vi "Write Config Unitest.vi"(8 "error in (no error)":errorcluster, 11 "main ref":T1) -> (0 "error out":errorcluster)   [LabVIEW 2025]
uses:
  v06/controls/LAB-IQ UI Data.ctl
  Traction Loop/Traction Receipe Enum.ctl
  Config file  FGV Unitest enum.ctl
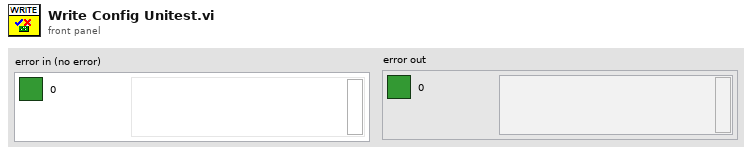
[diagram p1: front panel]
types:
  T1 = typedef "LAB-IQ UI Data.ctl" = cluster{"Main Home Screen":cluster{"GUI":refnum<vi>, "Platform Settings":refnum<vi>, "Configure":refnum<vi>, "Home":refnum<vi>, "EXIT":refnum<vi>, "service 2":refnum<vi>, "MainPage":refnum<vi>, "Analysis":refnum<vi>}, "Platform Settings":cluster{"mm/s  Surge":refnum<vi>, "Drive Error":refnum<vi>, "Disable Axis Jog Soft Limits":refnum<vi>, "mm/s  Sway":refnum<vi>, "Sway and Surge COM Status":refnum<vi>, "Heave COM Status":refnum<vi>, "Enable Platform":refnum<vi>, "Surge Forward Main":refnum<vi>, "Sway Right Main":refnum<vi>, "Sway Left Main":refnum<vi>, "Heave Down Main":refnum<vi>, "Heave Up main":refnum<vi>, "mm/s Heave":refnum<vi>, "mm/sec":refnum<vi>, "mm":refnum<vi>, "Surge Backward Main":refnum<vi>}, "Analysis Screen":cluster{"Analysis Home":refnum<vi>, "Surface Analysis":refnum<vi>, "Imaging":refnum<vi>, "Image Analysis":refnum<vi>, "Post Analysis":refnum<vi>}, "Config Screen":cluster{"Select Load Head":refnum<vi>, "Notes :":refnum<vi>, "FILE":refnum<vi>, "Sample ID :":refnum<vi>, "Operator ID :":refnum<vi>, "Operator Name :":refnum<vi>, "Auto":refnum<vi>}, "Motion Module":cluster{"zNL":refnum<vi>, "NL disp":refnum<vi>, "Rotary Tab":refnum<vi>, "Motion Direction:  3":refnum<vi>, "E.Velocity 2":refnum<vi>, "e.v/ssr 2":refnum<vi>, "Enter Fixed E.Velocity 2":refnum<vi>, "Enter Final SRR 2":refnum<vi>, "Enter initial SRR 2":refnum<vi>, "Enter Fixed SRR 2":refnum<vi>, "Enter the Final E.Velocity (m/s) 2":refnum<vi>, "Enter initial E.Velocity (m/s) 2":refnum<vi>, "Final Speed (RPM) 3":refnum<vi>, "Initial Speed (RPM) 2":refnum<vi>, "Enter the Final Velocity (m/s) 3":refnum<vi>, "Enter initial Velocity (m/s)  3":refnum<vi>, "Ramp Up 2":refnum<vi>, "TEST SELECTION":refnum<vi>, "SPEED SELECTION : ":refnum<vi>, "Angular Oscillation Set":refnum<vi>, "Traction":refnum<vi>, "Step Speed":refnum<vi>, "StepTable For Load-Speed":refnum<vi>, "StepTable For Speed":refnum<vi>, "Surge Forward MM":refnum<vi>, "Surge Backward MM":refnum<vi>, "M3 Image":refnum<vi>, "String 39":refnum<vi>, "Sway Left MM":refnum<vi>, "Sway Right MM":refnum<vi>, "Disable Axis Jog Soft Limits":refnum<vi>, "mm":refnum<vi>, "Heave Down MM":refnum<vi>, "Heave Up MM":refnum<vi>, "Wear Track Diameter (mm)":refnum<vi>, "Set WTD":refnum<vi>, "HomeScratch":refnum<vi>, "HomeRot":refnum<vi>, "PlaceModule":refnum<vi>, "Enter the Angle (Deg)":refnum<vi>, "Enter the Frequency (Hz)":refnum<vi>, "Motion Mode:":refnum<vi>, "LR Sway":refnum<vi>, "Rot Hor":refnum<vi>, "Scratch":refnum<vi>, "LR Cam":refnum<vi>, "MMBack":refnum<vi>, "MMNext":refnum<vi>, "Rot Ver":refnum<vi>, "Rotary Module Selection":refnum<vi>, "calculate rotary":refnum<vi>, "SPEED SELECTION : rotary":refnum<vi>, "Import 2":refnum<vi>, "Save 2":refnum<vi>, "File Path :  2":refnum<vi>, "String 45":refnum<vi>, "StepTable For Speed 3":refnum<vi>, "Enter the Speed(mm/sec)":refnum<vi>, "Enter the Speed(RPM)":refnum<vi>, "Enter Scratch Speed (mm/s):":refnum<vi>, "SwaySpeed Set":refnum<vi>, "Scartch Offset":refnum<vi>, "Motion type:":refnum<vi>, "HomeScratch 2":refnum<vi>, "Enter Scratch length (mm):":refnum<vi>, "Wear Track Diameter":refnum<vi>, "Rotary Speed Exced":refnum<vi>, "Scratch Mode":refnum<vi>, "No of Scratch":refnum<vi>}, "Environmental control":cluster{"Humidity  Status  3":refnum<vi>, "Low Temp  Status  2":refnum<vi>, "TK4 status 2":refnum<vi>, "Stage Temperature":refnum<vi>, "Sample Temperature":refnum<vi>, "Humidity (Amb)":refnum<vi>, "Clear List":refnum<vi>, "Add to list":refnum<vi>, "Wear":refnum<vi>, "Vibration":refnum<vi>, "Humidity (Chamber)":refnum<vi>, "Temperature (Chamber)":refnum<vi>, "ECR ":refnum<vi>, "Temperature (Amb)":refnum<vi>, "Microphone":refnum<vi>, "Acoustic Emission 3":refnum<vi>, "SNext":refnum<vi>, "APBack":refnum<vi>, "Enter the Temperature (°C):":refnum<vi>, "Enter the Stage \nTemperature (°C):":refnum<vi>, "Enter the Humidity (%Rh):":refnum<vi>, "Low Temp":refnum<vi>, "High Temp":refnum<vi>, "Humidity":refnum<vi>, "Sensors Picked":refnum<vi>}, "About Screen":cluster{"Password":refnum<vi>, "Home Service":refnum<vi>, "Advanced Setting":refnum<vi>, "About Tab":refnum<vi>, "ECR Port:":refnum<vi>, "Ramp Port:":refnum<vi>, "Installation/Replacement completed":refnum<vi>, "Loahead":refnum<vi>, "Heave and Surge COM Port:":refnum<vi>, "Sway COM Port:":refnum<vi>, "Temp Modbus:":refnum<vi>, "Humidity Port:":refnum<vi>, "Edit Gain Constants":refnum<vi>, "Save Gain Constants":refnum<vi>}, "Main Screen":cluster{"Main Screen Tab":refnum<vi>, "Angle and Frequency":refnum<vi>, "Stroke (mm)":refnum<vi>, "Angle (Deg)":refnum<vi>, "Main Speed Tab":refnum<vi>, "MTM MOTOR DISPLAY":refnum<vi>, "Disc Speed (m/sec)":refnum<vi>, "Ball Speed (m/sec)":refnum<vi>, "Disc Speed (RPM)":refnum<vi>, "Ball Speed (RPM)":refnum<vi>, "SPEED TAB":refnum<vi>, "Speed (m/sec)":refnum<vi>, "Set Speed (m/sec)":refnum<vi>, "Speed (RPM)":refnum<vi>, "Set Speed":refnum<vi>, "Time Tab":refnum<vi>, "Time ( HH:MM:SS ) 2":refnum<vi>, "Test Duration":refnum<vi>, "Test Duration 4":refnum<vi>, "TEST CYCLE":refnum<vi>, "TOTAL CYCLES":refnum<vi>, "Set Load (N)":refnum<vi>, "Temp Tabs":refnum<vi>, "Heater":refnum<vi>, "TK4 status":refnum<vi>, "ChamberTemp":refnum<vi>, "SetTmp":refnum<vi>, "Controller  Status":refnum<vi>, "ChamberTemp 2":refnum<vi>, "SetTmp 2":refnum<vi>, "Controller  Status 2":refnum<vi>, "ChamberTemp 3":refnum<vi>, "SetTmp 3":refnum<vi>, "Cooling":refnum<vi>, "Load Communication":refnum<vi>, "Ambient \nTemperature":refnum<vi>, "HumCOMStatus":refnum<vi>, "Ambient\n Humidity":refnum<vi>, "Freq (Hz)":refnum<vi>, "Load En":refnum<vi>, "NLt":refnum<vi>, "zNL 2":refnum<vi>, "Humidity On":refnum<vi>, "humidity disp":refnum<vi>, "Set Humidity":refnum<vi>, "NL disp 2":refnum<vi>, "Humidity On 2":refnum<vi>, "humidity disp 2":refnum<vi>, "Set Humidity 2":refnum<vi>, "NL disp 3":refnum<vi>, "AppLoadSeq scratch":refnum<vi>, "Stop Scratch":refnum<vi>, "ClrLog":refnum<vi>, "Trip Log":refnum<vi>, "STOP":refnum<vi>, "Start Test":refnum<vi>, "Test status":refnum<vi>, "AR Led":refnum<vi>, "Data":refnum<vi>, "Health":refnum<vi>, "Sway COM Status":refnum<vi>, "Heave COM Status":refnum<vi>, "Grp Tab":refnum<vi>, "Sub Graph":refnum<vi>, "SD (mm)":refnum<vi>, "Siliding distance Reset Graph":refnum<vi>, "SDGp":refnum<vi>, "Humidity Reset Graph":refnum<vi>, "HumrGp":refnum<vi>, "Acoustic Emission (mV)":refnum<vi>, "Aqucostic Reset Graph":refnum<vi>, "gACQUOS":refnum<vi>, "ECR RESET":refnum<vi>, "ECR":refnum<vi>, "Temperature Reset":refnum<vi>, "Acoustic Emission (mV) 2":refnum<vi>, "Aqucostic Reset Graph 2":refnum<vi>, "gACQUOS 2":refnum<vi>, "ECR RESET 2":refnum<vi>, "ECR 2":refnum<vi>, "Temperature Reset 2":refnum<vi>, "Temperature (deg c)":refnum<vi>, "Speed Reset Graph":refnum<vi>, "Speed Tab":refnum<vi>, "MTM DISC  SPEED":refnum<vi>, "MTM BALL SPEED":refnum<vi>, "speed mm/sec":refnum<vi>, "Hymidity":refnum<vi>, "Humidity Disable trip":refnum<vi>, "CoF Trip  2":refnum<vi>, "Depth Trip":refnum<vi>, "Weart Deapth":refnum<vi>, "Depth Reset Graph":refnum<vi>, "Weart":refnum<vi>, "Depthz":refnum<vi>, "Depth (µm)":refnum<vi>, "WearGp":refnum<vi>, "NL Trip 2":refnum<vi>, "Load pid":refnum<vi>, "Load Disable Trip":refnum<vi>, "Load Reset Graph":refnum<vi>, "NL Display 4":refnum<vi>, "Main Chart 3":refnum<vi>, "BACK":refnum<vi>, "Depth Trip 2":refnum<vi>, "COF TRIP ":refnum<vi>, "Friction Force (N)":refnum<vi>, "FF Reset Graph":refnum<vi>, "FF Disable Trip":refnum<vi>, "FF TRIP":refnum<vi>, "COF Disable Trip":refnum<vi>, "COF Reset Graph":refnum<vi>, "Start Test Temp":refnum<vi>, "zFF":refnum<vi>, "Friction Force (N) Graph":refnum<vi>, "Coefficient of Friction":refnum<vi>, "Scratch Start Test":refnum<vi>, "FF Tab":refnum<vi>, "Cyclic Friction Force (N)":refnum<vi>, "CZ FF":refnum<vi>, "Cyclic Friction Force (N) Graph":refnum<vi>, "Cyclic Coefficient of Friction":refnum<vi>, "Cyclic FF TRIP":refnum<vi>, "Cyclic FF Disable Trip":refnum<vi>, "cyclic COF Disable Trip":refnum<vi>, "cyclic COF TRIP":refnum<vi>, "cyclic COF Reset Graph":refnum<vi>, "Cyclic FF Reset Graph":refnum<vi>, "Test Trip":refnum<vi>, "Multi Scratch Pass":refnum<vi>, "Scratch Start Recording":refnum<vi>, "Coefficient of Friction 2":refnum<vi>, "Acoustic Emission":refnum<vi>, "Friction Force (N) 2":refnum<vi>, "Depth (Microns)":refnum<vi>, "Normal Load ( N )":refnum<vi>}, "Loading":cluster{"Indentation":refnum<vi>, "Reference Sample":refnum<vi>, "Load Cell Communication Slide":refnum<vi>, "com 3":refnum<vi>, "com":refnum<vi>, "DecaForce COM Status":refnum<vi>, "Update":refnum<vi>, "Clear 3":refnum<vi>, "seq":refnum<vi>, "Stribeck table":refnum<vi>, "Stribeck Table  For loading":refnum<vi>, "Loading Mode":refnum<vi>, "Enter the Final Load (N)":refnum<vi>, "Enter the CoF Trip":refnum<vi>, "Enter the Friction Force Trip":refnum<vi>, "Enter the Normal load Trip":refnum<vi>, "Enter the Load  (N)":refnum<vi>, "KiloForce":refnum<vi>, "DecaForce ":refnum<vi>, "MicroForce":refnum<vi>, "LHBack":refnum<vi>, "LHNext":refnum<vi>, "Enter the Loading Rate (N/min)":refnum<vi>, "Message":refnum<vi>, "Warning 2":refnum<vi>, "SSP 0.75":refnum<vi>, "SSP 0.5":refnum<vi>, "SSP 0.3":refnum<vi>, "Warning":refnum<vi>, "gui GIF":refnum<vi>, "Communication is established":refnum<vi>, "AppLoad 4":refnum<vi>, "Multipoint":refnum<vi>, "Load Selection":refnum<vi>}, "PID":cluster{"Ramp":refnum<vi>, "Vertical load (N)":refnum<vi>, "apply load":refnum<vi>, "apply load 2":refnum<vi>, "Enter ByPass Load":refnum<vi>, "Bypass Load":refnum<vi>, "gFF Rot":refnum<vi>}, "Config Parameters":cluster{"Tab Control 3":refnum<vi>, "Tab Control 19":refnum<vi>, "SAMPLES":refnum<vi>, "Re-initilaize":refnum<vi>, "Filter ON/OFF":refnum<vi>, "TracHomeSurgeOffsetCounts 10MM":refnum<vi>, "TracHomeSwayOffsetCounts 10MM":refnum<vi>, "Acoustic Emission:":refnum<vi>, "Apply Filter (FF)":refnum<vi>, "Filter% 2":refnum<vi>, "Apply Filter (Load)":refnum<vi>, "Filter% ":refnum<vi>, "Sway distance (mm)":refnum<vi>, "Surge distance (mm)":refnum<vi>, "DataSavingLoopDelay(ms)":refnum<vi>, "SAVE 2":refnum<vi>, "Enter Distance":refnum<vi>, "Sway Counts:":refnum<vi>, "Distance (mm): 3":refnum<vi>, "Surge Counts:":refnum<vi>, "Distance (mm): 2":refnum<vi>, "Distance (mm):":refnum<vi>, "Heave Counts:":refnum<vi>, "LRMHomeSurgeOffsetCounts":refnum<vi>, "LRMHomeSwayOffsetCounts":refnum<vi>, "TracHomeSurgeOffsetCounts 20MM":refnum<vi>, "TracHomeSwayOffsetCounts 20MM":refnum<vi>, "RotHomeSwayOffsetCounts":refnum<vi>, "RotHomeSurgeOffsetCounts":refnum<vi>, "Heave distance":refnum<vi>, "Zmm":refnum<vi>, "Heave Pulses/mm":refnum<vi>, "Surge Pulses/mm":refnum<vi>, "Sway Pulses/mm":refnum<vi>, "Heave Pitch":refnum<vi>, "Surge Pitch":refnum<vi>, "Sway Pitch":refnum<vi>, "Heave PPR":refnum<vi>, "Surge PPR":refnum<vi>, "Sway PPR":refnum<vi>, "Tab Control 5":refnum<vi>, "Tab Control 14":refnum<vi>, "Tab Control 26":refnum<vi>, "AE":refnum<vi>, "Heave Loop Delay":refnum<vi>, "Heave PID Speed":refnum<vi>, "Surge Jog Speed":refnum<vi>, "Heave Jog Speed":refnum<vi>, "Sway Loop Delay":refnum<vi>, "Sway PID Speed":refnum<vi>, "Sway Jog Speed":refnum<vi>, "DEPTH TRIP VALUE":refnum<vi>, "LOAD TRIP VALUE":refnum<vi>, "DEPTH TRIP   ENABLE":refnum<vi>, "LOAD TRIP  ENABLE":refnum<vi>, "CYCLIC FF TRIP VALUE":refnum<vi>, "FF TRIP VALUE":refnum<vi>, "CYCLIC CoF TRIP VALUE":refnum<vi>, "COF TRIP VALUE":refnum<vi>, "CYCLIC COF TRIP  ENABLE":refnum<vi>, "CYCLIC FF TRIP  ENABLE":refnum<vi>, "FF TRIP  ENABLE":refnum<vi>, "COF TRIP  ENABLE":refnum<vi>, "JOG TRIP LOAD VALUE (N)":refnum<vi>, "Rotary Vertical":refnum<vi>, "Traction":refnum<vi>, "Scratch":refnum<vi>, "LRM CAM":refnum<vi>, "Sway LRM":refnum<vi>, "Rotary Horizontal":refnum<vi>, "SURGE SPEED":refnum<vi>, "SURGE BACKWARD COUNT":refnum<vi>, "SURGE FORWARD COUNT":refnum<vi>, "Start Button":refnum<vi>}, "Loading Com Port":cluster{"ClearAll":refnum<vi>, "Mz(Nm)":refnum<vi>, "My(Nm)":refnum<vi>, "Mx(Nm)":refnum<vi>, "Save Dwell":refnum<vi>, "Acq Delay (ms)":refnum<vi>, "Burst Delay (ms)":refnum<vi>, "model":refnum<vi>, "SN":refnum<vi>, "FFx(N)":refnum<vi>, "Sensor IP":refnum<vi>, "Port":refnum<vi>, "FFy(N)":refnum<vi>, "Load(N)":refnum<vi>, "delete Handle":refnum<vi>, "Create Handle":refnum<vi>, "ft_data":refnum<vi>, "ft_range":refnum<vi>, "ft_data 2":refnum<vi>, "stop 6":refnum<vi>, "running_flag":refnum<vi>, "ft_udp_handle":refnum<vi>, "get-data-return":refnum<vi>, "get-range-return":refnum<vi>, "zero-return":refnum<vi>, "filter-return":refnum<vi>, "initial-return":refnum<vi>, "deleteHandle-result":refnum<vi>, "Load Cell Temp":refnum<vi>, "Load Cell":refnum<vi>, "ZeroAll":refnum<vi>, "FORCE (N)":refnum<vi>, "TORQUE (N-m)":refnum<vi>, "Load Cell Link":refnum<vi>}, "Heave AND Surge":cluster{"SURGE POSE":refnum<vi>, "error out Read":refnum<vi>, "HEAVE POSE":refnum<vi>, "State":refnum<vi>, "Homed":refnum<vi>, "Sequence ID":refnum<vi>, "error out Write":refnum<vi>, "faultCode":refnum<vi>, "Ack ID":refnum<vi>, "SPEED":refnum<vi>, "Distance":refnum<vi>, "Mode Command":refnum<vi>, "Heave and Surge Read":refnum<vi>, "Read Heave Temp":refnum<vi>, "Spare 15":refnum<vi>, "Spare 14":refnum<vi>, "Spare 13":refnum<vi>, "Spare 12":refnum<vi>, "Spare 11":refnum<vi>, "Spare 10":refnum<vi>, "Spare 9":refnum<vi>, "Spare 8":refnum<vi>, "Spare 7":refnum<vi>, "Spare 4":refnum<vi>, "Spare 3":refnum<vi>, "Spare 2":refnum<vi>, "Humidity":refnum<vi>, "Temp":refnum<vi>, "Node Id":refnum<vi>, "Spare 1":refnum<vi>, "SPARE 4":refnum<vi>, "SPARE 3":refnum<vi>, "SPARE 2":refnum<vi>, "SPARE 1":refnum<vi>, "fwMajor":refnum<vi>, "fwMinor":refnum<vi>, "Manual Write":refnum<vi>, "Heave and Surge Write":refnum<vi>, "SPARE 5":refnum<vi>, "Reserved ":refnum<vi>, "SPARE 8":refnum<vi>, "SPARE 6":refnum<vi>, "SPARE 7":refnum<vi>, "SPARE 17":refnum<vi>, "SPARE 16":refnum<vi>, "SPARE 15":refnum<vi>, "SPARE 14":refnum<vi>, "SPARE 13":refnum<vi>, "SPARE 12":refnum<vi>, "SPARE 11":refnum<vi>, "SPARE 10":refnum<vi>, "SPARE 9":refnum<vi>, "System UPTIME":refnum<vi>, "Missed Packets":refnum<vi>, "faultCode Surge Right":refnum<vi>, "faultCode Surge Left":refnum<vi>, "faultCode Heave":refnum<vi>, "UPLINK HEAVE":refnum<vi>, "DOWNLINK HEAVE":refnum<vi>}, "New PID LOGIC":cluster{"Fine Tune Zone":refnum<vi>, "PID SDelay":refnum<vi>, "Max_pos_limit":refnum<vi>, "Min_pos_limit":refnum<vi>, "i_limit":refnum<vi>, "pct_scale":refnum<vi>, "Deadband":refnum<vi>, "Kd":refnum<vi>, "Ki":refnum<vi>, "Kp":refnum<vi>, "Current Position":refnum<vi>, "Set Load":refnum<vi>, "Current Load":refnum<vi>, "Pulse delta":refnum<vi>, "Init Step":refnum<vi>, "Max Step Linit":refnum<vi>, "min_deadband_floor":refnum<vi>, "dynamic_spindle_noise_scalar":refnum<vi>, "min_finetune_floor":refnum<vi>, "filter_alpha":refnum<vi>, "PID":refnum<vi>}, "SWAY ":cluster{"fwMajor":refnum<vi>, "Homed":refnum<vi>, "Rotary POSE":refnum<vi>, "State":refnum<vi>, "SWAY POSE":refnum<vi>, "Ack ID":refnum<vi>, "faultCode":refnum<vi>, "Node Id":refnum<vi>, "fwMinor":refnum<vi>, "Spare 6":refnum<vi>, "Spare 5":refnum<vi>, "Spare 4":refnum<vi>, "Spare 3":refnum<vi>, "Spare 2":refnum<vi>, "Spare 1":refnum<vi>, "Spare 7":refnum<vi>, "SPARE  5":refnum<vi>, "error out Write  SWAY ":refnum<vi>, "error out Read SWAY ":refnum<vi>, "Manual Write SWAY ":refnum<vi>, "SWAY WRITE":refnum<vi>, "SPARE  4":refnum<vi>, "SPARE  3":refnum<vi>, "SPARE 2":refnum<vi>, "SPARE 1":refnum<vi>, "Spare 15":refnum<vi>, "Spare 14":refnum<vi>, "Spare 13":refnum<vi>, "Spare 12":refnum<vi>, "Spare 11":refnum<vi>, "Spare 9":refnum<vi>, "Spare 8":refnum<vi>, "SPEED":refnum<vi>, "Distance":refnum<vi>, "Mode Command":refnum<vi>, "Sequence ID":refnum<vi>, "SWAY READ":refnum<vi>, "Spare 10":refnum<vi>, "Read SWAY Temp":refnum<vi>, "faultCode Sway ":refnum<vi>, "Missed Packets":refnum<vi>, "System UPTIME sway":refnum<vi>, "SPARE 6":refnum<vi>, "SPARE 7":refnum<vi>, "SPARE 9":refnum<vi>, "SPARE 11":refnum<vi>, "SPARE 10":refnum<vi>, "SPARE 8":refnum<vi>, "SPARE 13":refnum<vi>, "SPARE 12":refnum<vi>, "SPARE 17":refnum<vi>, "SPARE 16":refnum<vi>, "SPARE 15":refnum<vi>, "SPARE 14":refnum<vi>, "Reserved":refnum<vi>, "faultCode Rotary":refnum<vi>, "UPLINK SWAY":refnum<vi>, "DOWNLINK SWAY":refnum<vi>}, "Analysis Screen":cluster{"Analysis Home":refnum<vi>, "Refresh 2":refnum<vi>, "MEAN 4":refnum<vi>, "SD 4":refnum<vi>, "VARIANCE 4":refnum<vi>, "MEAN  3":refnum<vi>, "SD  3":refnum<vi>, "VARIANCE  3":refnum<vi>, "MEAN 2":refnum<vi>, "SD  2":refnum<vi>, "VARIANCE 2":refnum<vi>, "MEAN":refnum<vi>, "SD":refnum<vi>, "VARIANCE":refnum<vi>, "File 4 Discription":refnum<vi>, "OPEN 4":refnum<vi>, "File Name 4":refnum<vi>, "OPEN 3":refnum<vi>, "File 3 Discription":refnum<vi>, "File Name 3":refnum<vi>, "Y-AXIS":refnum<vi>, "X-AXIS":refnum<vi>, "XY Graph":refnum<vi>, "File Name 2":refnum<vi>, "File Name 1":refnum<vi>, "OPEN 2":refnum<vi>, "OPEN 1":refnum<vi>, "File 1 Discription ":refnum<vi>, "File 2 Discription":refnum<vi>, "Export":refnum<vi>, "File Format":refnum<vi>}, "Traction":cluster{"faultCode Traction 2":refnum<vi>, "faultCode Traction 1":refnum<vi>, "Missed Packets":refnum<vi>, "System UPTIME Traction":refnum<vi>, "SPARE 17":refnum<vi>, "SPARE 16":refnum<vi>, "SPARE 15":refnum<vi>, "SPARE 14":refnum<vi>, "SPARE 13":refnum<vi>, "SPARE 12":refnum<vi>, "SPARE 11":refnum<vi>, "SPARE 10":refnum<vi>, "SPARE 9":refnum<vi>, "SPARE 8":refnum<vi>, "SPARE 7":refnum<vi>, "SPARE 6":refnum<vi>, "Reserved":refnum<vi>, "SPARE  5":refnum<vi>, "Manual Write TRACTION":refnum<vi>, "TRACTION WRITE":refnum<vi>, "SPARE  4":refnum<vi>, "SPARE  3":refnum<vi>, "SPARE 2":refnum<vi>, "SPARE 1":refnum<vi>, "Spare 7":refnum<vi>, "Spare 6":refnum<vi>, "Spare 5":refnum<vi>, "Spare 4":refnum<vi>, "Spare 2":refnum<vi>, "Spare 1":refnum<vi>, "Node Id":refnum<vi>, "Read TRACTION Temp":refnum<vi>, "fwMinor":refnum<vi>, "fwMajor":refnum<vi>, "faultCode":refnum<vi>, "TRACTION POSE":refnum<vi>, "TRACTION POSE 2":refnum<vi>, "Homed":refnum<vi>, "State":refnum<vi>, "Ack ID":refnum<vi>, "SPEED":refnum<vi>, "Distance":refnum<vi>, "Mode Command":refnum<vi>, "Sequence ID":refnum<vi>, "error out Read TRACTION":refnum<vi>, "error out Write  TRACTION":refnum<vi>, "TRACTION READ":refnum<vi>, "Spare 3":refnum<vi>, "Downlink traction":refnum<vi>, "Uplink Traction":refnum<vi>}, "Traction reciepe":cluster{"SRR Sweep Range (%) Stribeck":refnum<vi>, "Traction Receipe":refnum<vi>, "Total Execution Time":refnum<vi>, "Total Steps":refnum<vi>, "Duration / Step (s)  Stribeck":refnum<vi>, "STRIBECK Fixed SRR List (%)":refnum<vi>, "Duration / Step (s) Traction":refnum<vi>, "SRR Sweep Range (%) traction":refnum<vi>, "Rolling Speed (mm/s)":refnum<vi>, "Temperature Stages (°C)":refnum<vi>, "Ball Load (N)":refnum<vi>, "Lubricant Name":refnum<vi>, "Profile File Name":refnum<vi>, "SET entrainment Velocity":refnum<vi>, "Test Array Size":refnum<vi>, "SRR INDEX [ STRIBECK]":refnum<vi>, "Stribeck Size":refnum<vi>, "SET SRR":refnum<vi>, "ELAPSED TIMER ":refnum<vi>, "BALL SET RPM":refnum<vi>, "DISC SET RPM":refnum<vi>, "SET LOAD":refnum<vi>, "TEMPERATURE READ":refnum<vi>, "SET TEMPERATURE":refnum<vi>, "Traction Size":refnum<vi>, "DISC SPEED (rpm)":refnum<vi>, "BALL SPEED (rpm)":refnum<vi>, "BALL WEAR TRACK":refnum<vi>, "DISC WEARTRACK":refnum<vi>, "SRR INDEX [ TRACTION]":refnum<vi>, "Start Index Type":refnum<vi>, "Enum - Menu":refnum<vi>, "Ball (mm/sec)":refnum<vi>, "Disc (mm/sec)":refnum<vi>, "Traction Receipe Update Details":refnum<vi>}, "Traction Control":cluster{"HomeTraction":refnum<vi>, "Demo Mode Display":refnum<vi>, "Traction Message":refnum<vi>, "Traction Step Update Details":refnum<vi>, "Main Tab sequence for selection":refnum<vi>, "Ramp Tab":refnum<vi>, "e.v/ssr":refnum<vi>, "Enter Fixed E.Velocity":refnum<vi>, "Enter Final SRR":refnum<vi>, "Enter initial SRR":refnum<vi>, "Enter Fixed SRR":refnum<vi>, "Enter the Final E.Velocity (m/s)":refnum<vi>, "Enter initial E.Velocity (m/s)":refnum<vi>, "Ball WTD":refnum<vi>, "E.Velocity":refnum<vi>, "Enter the Final Velocity (m/s)":refnum<vi>, "Enter initial Velocity (m/s)":refnum<vi>, "Ramp Up   Disc":refnum<vi>, "Initial DiscSpeed (RPM)":refnum<vi>, "Final Speed (RPM) Ball":refnum<vi>, "Final Speed (RPM)":refnum<vi>, "Initial Speed (RPM) Ball":refnum<vi>, "Enter the Final Velocity (m/s) Ball":refnum<vi>, "Enter initial Velocity (m/s) Ball":refnum<vi>, "Ramp Up":refnum<vi>, "ExceedBallSpeed step":refnum<vi>, "ExceedDiscSpeed":refnum<vi>, "BallSpeed Exceed Indication":refnum<vi>, "Apply":refnum<vi>, "SPEED SELECTION : MTM":refnum<vi>, "SPEED SELECTION : MTM 2":refnum<vi>, "TEST SELECTION (MTM)":refnum<vi>, "MTM Test Selection":refnum<vi>, "File Path Tab":refnum<vi>, "File Path String":refnum<vi>, "Save":refnum<vi>, "Save  2":refnum<vi>, "Import ":refnum<vi>, "File Path :":refnum<vi>, "Step Sequence Indication Tab":refnum<vi>, "Step Sequence Indication":refnum<vi>, "Calculate Step":refnum<vi>, "StepTable":refnum<vi>, "ExceedDiscSpeed  Cinstant Speed":refnum<vi>, "ExceedBallSpeed Constant":refnum<vi>, "TEST SELECTION (MTM) 2":refnum<vi>, "SPEED SELECTION : MTM 3":refnum<vi>, "MTM Test Selection 2":refnum<vi>, "Enter the Speed (m/sec): ":refnum<vi>, "Enter the Speed (m/sec):  2":refnum<vi>, "Enter the Speed (RPM):":refnum<vi>, "Lower Spped ":refnum<vi>, "Upper":refnum<vi>, "Enter the Speed (RPM):Ball":refnum<vi>, "Disc Motion Direction: ":refnum<vi>, "Ball Motion Direction :":refnum<vi>, "Motion Mode: ":refnum<vi>, "Wear Track Diameter (mm) ":refnum<vi>, "Disc Speed Indicator":refnum<vi>, "ExceedBallSpeed":refnum<vi>}, "Acquostic":cluster{"Last Config Rejected ":refnum<vi>, "rx command count":refnum<vi>, "Current Filter Id":refnum<vi>, "Isolated Gain":refnum<vi>, "DAQ Status":refnum<vi>, "error out":refnum<vi>, "error in (no error)":refnum<vi>, "Uplink Packet":refnum<vi>, "data out":refnum<vi>, "Downlink Packet":refnum<vi>, "Gains":refnum<vi>, "Manual Write Acquostic":refnum<vi>, "Acoustic Graphs":refnum<vi>}, "ABOUT":cluster{"version":refnum<vi>, "Operating System":refnum<vi>, "Version":refnum<vi>, "Workorder":refnum<vi>, "Runtime":refnum<vi>, "Instrument Serial":refnum<vi>, "Firmware Version":refnum<vi>, "Info":refnum<vi>}, "Temperature Port":cluster{"Temperature":refnum<vi>, "error out Temperature":refnum<vi>, "READ TEMPERATURE":refnum<vi>}}
  T2 = typedef "Config file  FGV Unitest enum.ctl" = enum16{"OPEN", "READ", "WRITE", "CLOSE"}
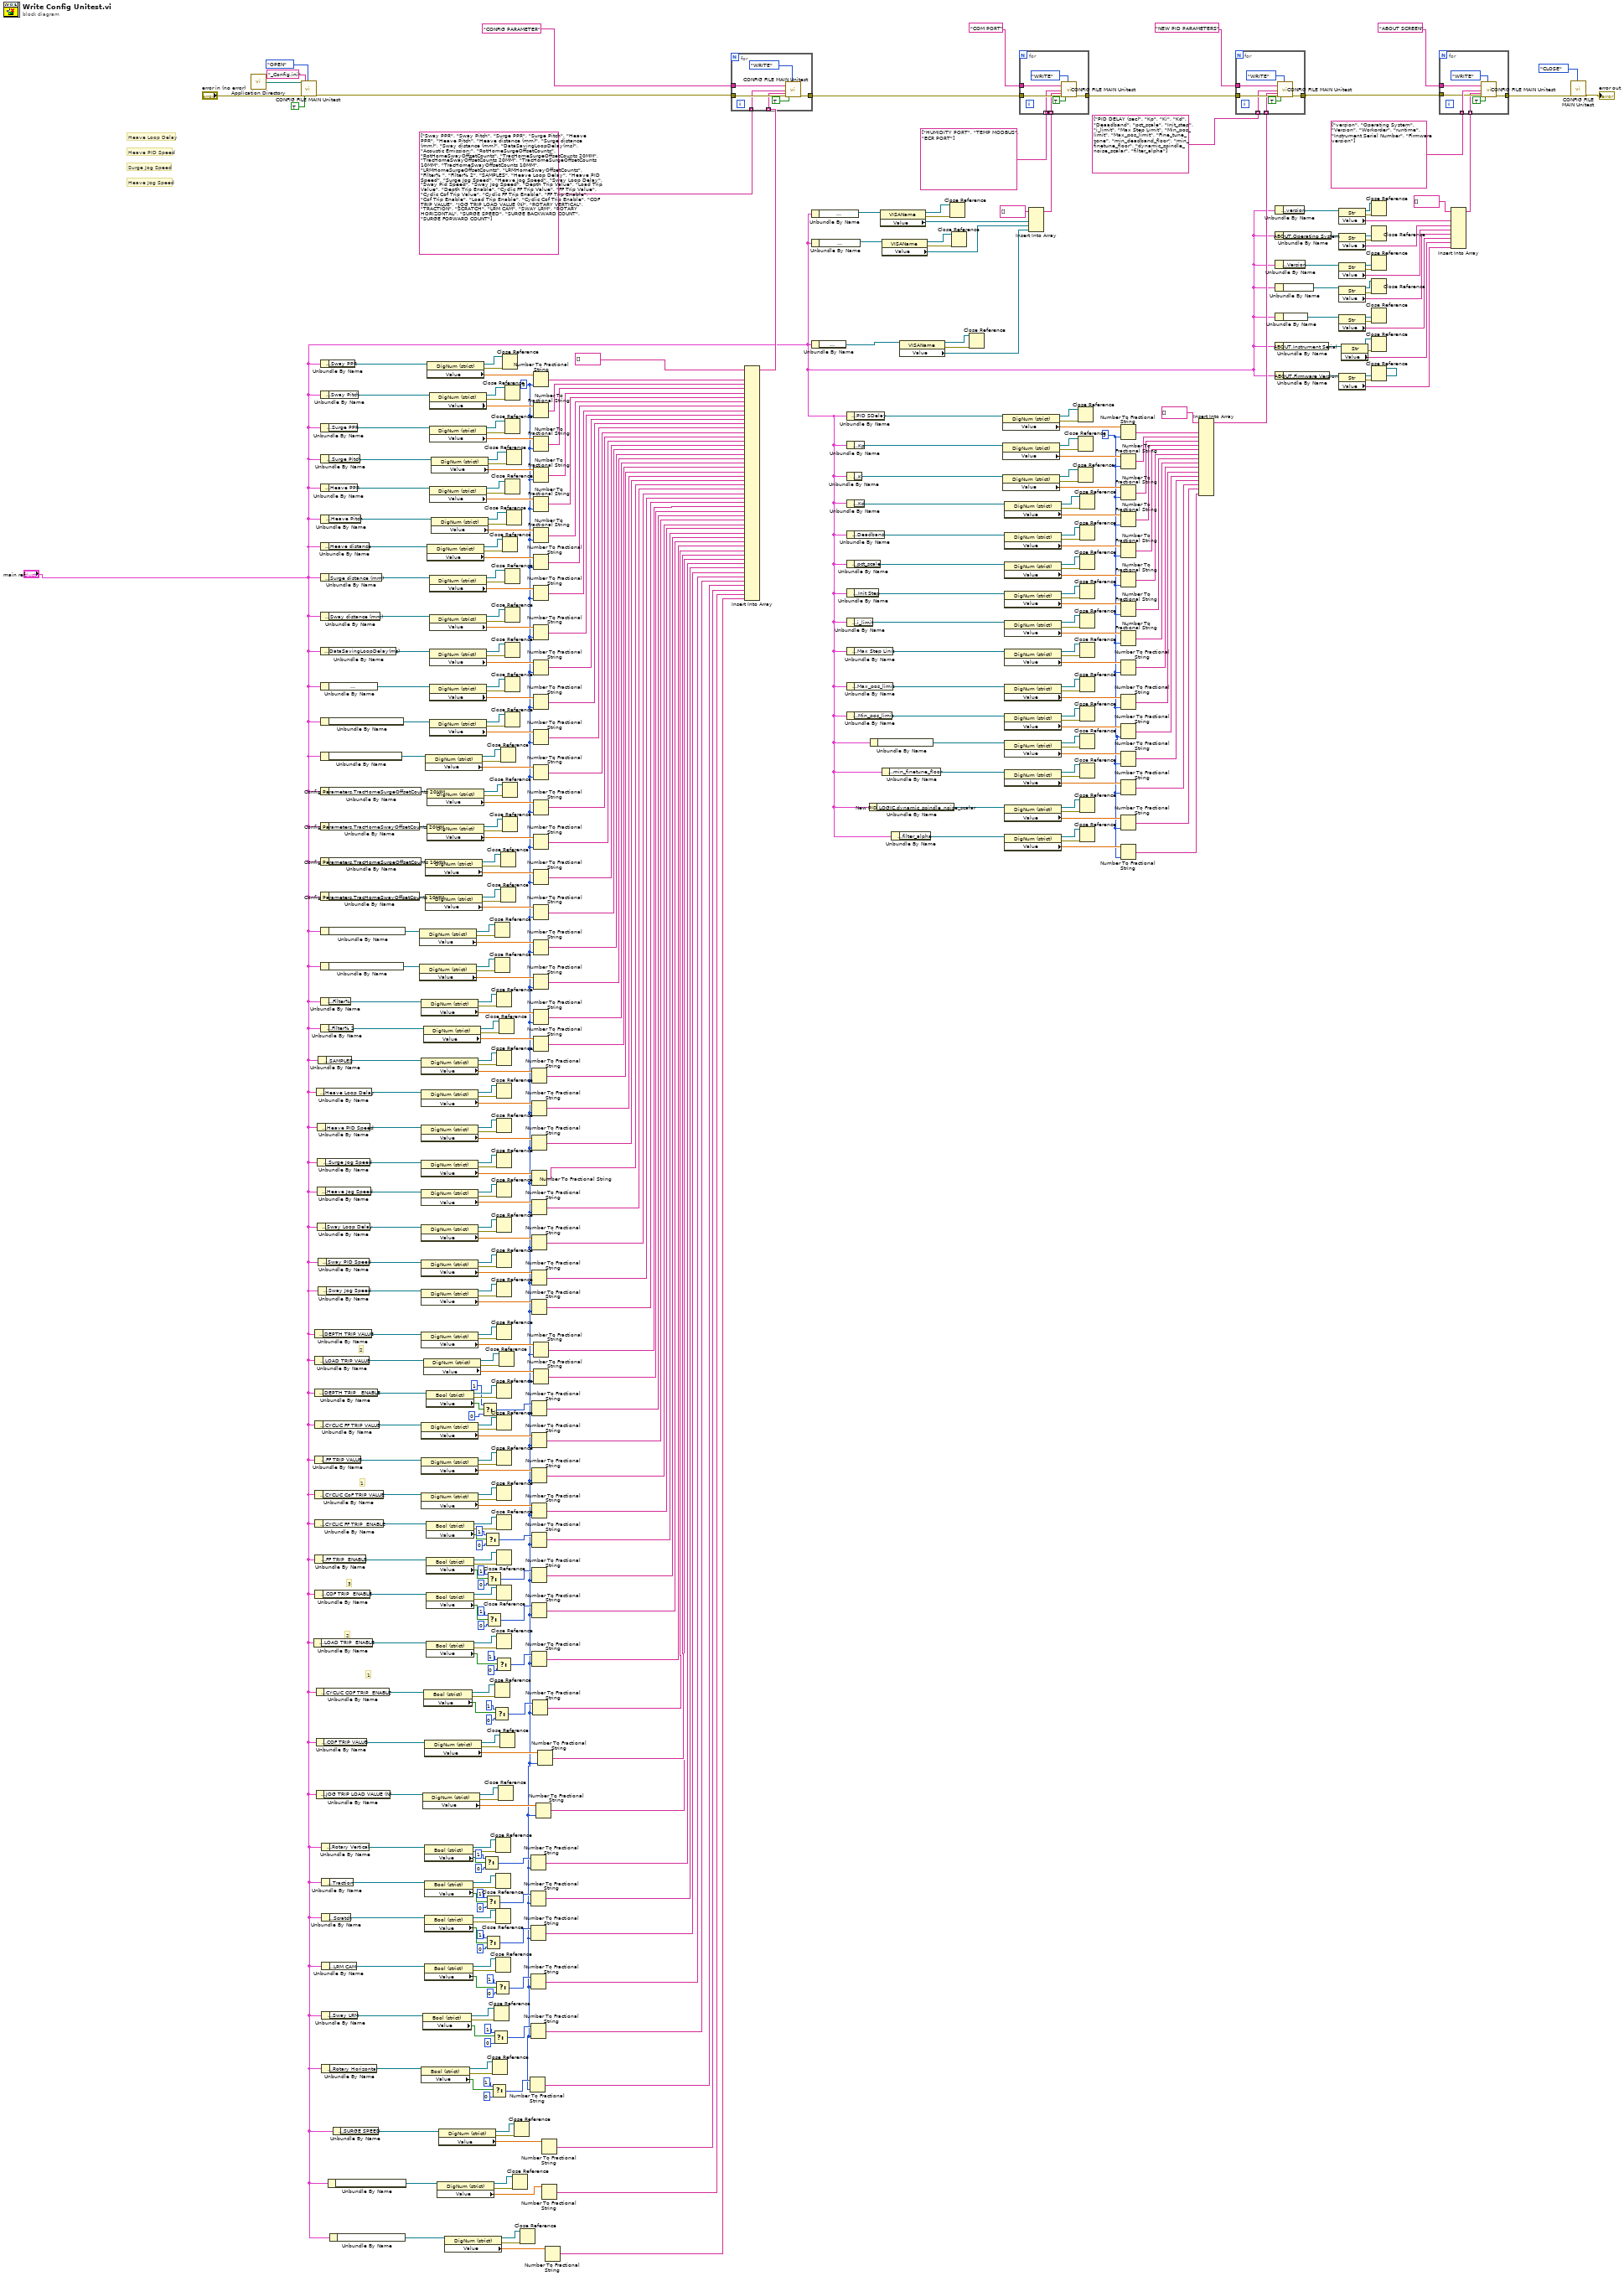
[diagram p0: block diagram]
diagram:
  w111 = i16 5 ("precision (6)")
  w60 = i16 5 ("precision (6)")
  # "3"
  # "2"
  # "2"
  # "1"
  # "1"
  # "Heave Jog Speed"
  # "Surge Jog Speed"
  # "Heave PID Speed"
  # "Heave Loop Delay"
  n1 = call <vilib>:"Application Directory.vi"() -> ("Application Directory"=w433:path)
  n2 = call "CONFIG FILE MAIN Unitest.vi"("File Path"=w433, "error in"="error in (no error)", "file name"="_Config.ini", "PARAMETER/CONFIG"=TRUE, "Config Enum"=Config_file__FGV_Unitest_enum."OPEN") -> ("error out"=w432:errorcluster)  [unwired: 13 in, 1 out]
  n3 = Unbundle By Name("main ref") -> ("Config Parameters.LOAD TRIP  ENABLE"=w171:refnum<vi>)
  n4 = Unbundle By Name("main ref") -> ("Config Parameters.DEPTH TRIP VALUE"=w175:refnum<vi>)
  n5 = Unbundle By Name("main ref") -> ("Config Parameters.LOAD TRIP VALUE"=w181:refnum<vi>)
  n6 = Unbundle By Name("main ref") -> ("Config Parameters.DEPTH TRIP   ENABLE"=w182:refnum<vi>)
  n7 = Unbundle By Name("main ref") -> ("Config Parameters.CYCLIC FF TRIP VALUE"=w189:refnum<vi>)
  n8 = Unbundle By Name("main ref") -> ("Config Parameters.FF TRIP VALUE"=w190:refnum<vi>)
  n9 = Unbundle By Name("main ref") -> ("Config Parameters.CYCLIC CoF TRIP VALUE"=w197:refnum<vi>)
  n10 = Unbundle By Name("main ref") -> ("Config Parameters.CYCLIC FF TRIP  ENABLE"=w198:refnum<vi>)
  n11 = Unbundle By Name("main ref") -> ("Config Parameters.FF TRIP  ENABLE"=w206:refnum<vi>)
  n12 = Unbundle By Name("main ref") -> ("Config Parameters.COF TRIP  ENABLE"=w201:refnum<vi>)
  n13 = Unbundle By Name("main ref") -> ("Config Parameters.CYCLIC COF TRIP  ENABLE"=w156:refnum<vi>)
  n14 = Unbundle By Name("main ref") -> ("Config Parameters.COF TRIP VALUE"=w134:refnum<vi>)
  n15 = Unbundle By Name("main ref") -> ("Config Parameters.JOG TRIP LOAD VALUE (N)"=w103:refnum<vi>)
  n16 = Unbundle By Name("main ref") -> ("Config Parameters.Heave Loop Delay"=w297:refnum<vi>)
  n17 = Unbundle By Name("main ref") -> ("Config Parameters.Heave PID Speed"=w296:refnum<vi>)
  n18 = Unbundle By Name("main ref") -> ("Config Parameters.Surge Jog Speed"=w289:refnum<vi>)
  n19 = Unbundle By Name("main ref") -> ("Config Parameters.Heave Jog Speed"=w288:refnum<vi>)
  n20 = Unbundle By Name("main ref") -> ("Config Parameters.Sway Loop Delay"=w210:refnum<vi>)
  n21 = Unbundle By Name("main ref") -> ("Config Parameters.SAMPLES"=w342:refnum<vi>)
  n22 = Unbundle By Name("main ref") -> ("Config Parameters.Sway PID Speed"=w217:refnum<vi>)
  n23 = Unbundle By Name("main ref") -> ("Config Parameters.Sway Jog Speed"=w218:refnum<vi>)
  n24 = Unbundle By Name("main ref") -> ("Config Parameters.Sway PPR"=w424:refnum<vi>)
  n25 = Unbundle By Name("main ref") -> ("Config Parameters.Sway Pitch"=w417:refnum<vi>)
  n26 = Unbundle By Name("main ref") -> ("Config Parameters.Surge PPR"=w409:refnum<vi>)
  n27 = Unbundle By Name("main ref") -> ("Config Parameters.Surge Pitch"=w416:refnum<vi>)
  n28 = Unbundle By Name("main ref") -> ("Config Parameters.Heave PPR"=w408:refnum<vi>)
  n29 = Unbundle By Name("main ref") -> ("Config Parameters.Heave Pitch"=w402:refnum<vi>)
  n30 = Unbundle By Name("main ref") -> ("Config Parameters.Heave distance"=w394:refnum<vi>)
  n31 = Unbundle By Name("main ref") -> ("Config Parameters.Surge distance (mm)"=w400:refnum<vi>)
  n32 = Unbundle By Name("main ref") -> ("Config Parameters.Sway distance (mm)"=w391:refnum<vi>)
  n33 = Unbundle By Name("main ref") -> ("Config Parameters.DataSavingLoopDelay(ms)"=w388:refnum<vi>)
  n34 = Unbundle By Name("main ref") -> ("Config Parameters.Acoustic Emission:"=w383:refnum<vi>)
  n35 = Unbundle By Name("main ref") -> ("Config Parameters.RotHomeSurgeOffsetCounts"=w380:refnum<vi>)
  n36 = Unbundle By Name("main ref") -> ("Config Parameters.RotHomeSwayOffsetCounts"=w375:refnum<vi>)
  n37 = Unbundle By Name("main ref") -> ("Config Parameters.TracHomeSurgeOffsetCounts 20MM"=w372:refnum<vi>)
  n38 = Unbundle By Name("main ref") -> ("Config Parameters.TracHomeSwayOffsetCounts 20MM"=w367:refnum<vi>)
  n39 = Unbundle By Name("main ref") -> ("Config Parameters.TracHomeSurgeOffsetCounts 10MM"=w361:refnum<vi>)
  n40 = Unbundle By Name("main ref") -> ("Config Parameters.TracHomeSwayOffsetCounts 10MM"=w366:refnum<vi>)
  n41 = Unbundle By Name("main ref") -> ("Config Parameters.LRMHomeSurgeOffsetCounts"=w355:refnum<vi>)
  n42 = Unbundle By Name("main ref") -> ("Config Parameters.LRMHomeSwayOffsetCounts"=w350:refnum<vi>)
  n43 = Unbundle By Name("main ref") -> ("Config Parameters.Filter%"=w349:refnum<vi>)
  n44 = Unbundle By Name("main ref") -> ("Config Parameters.Filter% 2"=w343:refnum<vi>)
  n45 = Unbundle By Name("main ref") -> ("Config Parameters.Rotary Vertical"=w75:refnum<vi>)
  n46 = Unbundle By Name("main ref") -> ("Config Parameters.Traction"=w67:refnum<vi>)
  n47 = Unbundle By Name("main ref") -> ("Config Parameters.Scratch"=w72:refnum<vi>)
  n48 = Unbundle By Name("main ref") -> ("Config Parameters.LRM CAM"=w76:refnum<vi>)
  n49 = Unbundle By Name("main ref") -> ("Config Parameters.Sway LRM"=w90:refnum<vi>)
  n50 = Unbundle By Name("main ref") -> ("Config Parameters.Rotary Horizontal"=w63:refnum<vi>)
  n51 = Unbundle By Name("main ref") -> ("Config Parameters.SURGE BACKWARD COUNT"=w46:refnum<vi>)
  n52 = Unbundle By Name("main ref") -> ("Config Parameters.SURGE FORWARD COUNT"=w45:refnum<vi>)
  n53 = Unbundle By Name("main ref") -> ("Config Parameters.SURGE SPEED"=w51:refnum<vi>)
  n54 = property class="DigNum (strict)"(reference=w355) -> (reference out=w356:refnum<vi>, error out=w354:errorcluster, "Value"=w353:dbl)  [unwired: 1 in]
  n55 = property class="DigNum (strict)"(reference=w350) -> (reference out=w357:refnum<vi>, error out=w351:errorcluster, "Value"=w352:dbl)  [unwired: 1 in]
  n56 = property class="DigNum (strict)"(reference=w349) -> (reference out=w346:refnum<vi>, error out=w348:errorcluster, "Value"=w347:dbl)  [unwired: 1 in]
  n57 = property class="DigNum (strict)"(reference=w342) -> (reference out=w339:refnum<vi>, error out=w341:errorcluster, "Value"=w340:dbl)  [unwired: 1 in]
  n58 = property class="DigNum (strict)"(reference=w297) -> (reference out=w300:refnum<vi>, error out=w298:errorcluster, "Value"=w299:dbl)  [unwired: 1 in]
  n59 = property class="DigNum (strict)"(reference=w296) -> (reference out=w293:refnum<vi>, error out=w295:errorcluster, "Value"=w294:dbl)  [unwired: 1 in]
  n60 = property class="DigNum (strict)"(reference=w289) -> (reference out=w292:refnum<vi>, error out=w290:errorcluster, "Value"=w291:dbl)  [unwired: 1 in]
  n61 = property class="DigNum (strict)"(reference=w288) -> (reference out=w285:refnum<vi>, error out=w287:errorcluster, "Value"=w286:dbl)  [unwired: 1 in]
  n62 = property class="DigNum (strict)"(reference=w210) -> (reference out=w213:refnum<vi>, error out=w211:errorcluster, "Value"=w212:dbl)  [unwired: 1 in]
  n63 = property class="DigNum (strict)"(reference=w217) -> (reference out=w214:refnum<vi>, error out=w216:errorcluster, "Value"=w215:dbl)  [unwired: 1 in]
  n64 = property class="DigNum (strict)"(reference=w218) -> (reference out=w221:refnum<vi>, error out=w219:errorcluster, "Value"=w220:dbl)  [unwired: 1 in]
  n65 = property class="DigNum (strict)"(reference=w175) -> (reference out=w178:refnum<vi>, error out=w176:errorcluster, "Value"=w177:dbl)  [unwired: 1 in]
  n66 = property class="DigNum (strict)"(reference=w189) -> (reference out=w186:refnum<vi>, error out=w188:errorcluster, "Value"=w187:dbl)  [unwired: 1 in]
  n67 = property class="DigNum (strict)"(reference=w190) -> (reference out=w193:refnum<vi>, error out=w191:errorcluster, "Value"=w192:dbl)  [unwired: 1 in]
  n68 = property class="DigNum (strict)"(reference=w197) -> (reference out=w194:refnum<vi>, error out=w196:errorcluster, "Value"=w195:dbl)  [unwired: 1 in]
  n69 = property class="Bool (strict)"(reference=w63) -> (reference out=w65:refnum<vi>, error out=w64:errorcluster, "Value"=w62:bool)  [unwired: 1 in]
  n70 = property class="DigNum (strict)"(reference=w103) -> (reference out=w105:refnum<vi>, error out=w104:errorcluster, "Value"=w106:dbl)  [unwired: 1 in]
  n71 = property class="Bool (strict)"(reference=w90) -> (reference out=w88:refnum<vi>, error out=w89:errorcluster, "Value"=w99:bool)  [unwired: 1 in]
  n72 = property class="DigNum (strict)"(reference=w343) -> (reference out=w338:refnum<vi>, error out=w344:errorcluster, "Value"=w345:dbl)  [unwired: 1 in]
  n73 = property class="DigNum (strict)"(reference=w181) -> (reference out=w185:refnum<vi>, error out=w180:errorcluster, "Value"=w179:dbl)  [unwired: 1 in]
  n74 = property class="Bool (strict)"(reference=w156) -> (reference out=w158:refnum<vi>, error out=w157:errorcluster, "Value"=w147:bool)  [unwired: 1 in]
  n75 = property class="DigNum (strict)"(reference=w134) -> (reference out=w132:refnum<vi>, error out=w133:errorcluster, "Value"=w131:dbl)  [unwired: 1 in]
  n76 = property class="Bool (strict)"(reference=w75) -> (reference out=w73:refnum<vi>, error out=w74:errorcluster, "Value"=w94:bool)  [unwired: 1 in]
  n77 = property class="Bool (strict)"(reference=w67) -> (reference out=w69:refnum<vi>, error out=w68:errorcluster, "Value"=w93:bool)  [unwired: 1 in]
  n78 = property class="Bool (strict)"(reference=w72) -> (reference out=w70:refnum<vi>, error out=w71:errorcluster, "Value"=w92:bool)  [unwired: 1 in]
  n79 = property class="Bool (strict)"(reference=w76) -> (reference out=w78:refnum<vi>, error out=w77:errorcluster, "Value"=w91:bool)  [unwired: 1 in]
  n80 = property class="DigNum (strict)"(reference=w375) -> (reference out=w374:refnum<vi>, error out=w376:errorcluster, "Value"=w377:dbl)  [unwired: 1 in]
  n81 = property class="DigNum (strict)"(reference=w361) -> (reference out=w359:refnum<vi>, error out=w362:errorcluster, "Value"=w363:dbl)  [unwired: 1 in]
  n82 = property class="DigNum (strict)"(reference=w366) -> (reference out=w358:refnum<vi>, error out=w365:errorcluster, "Value"=w364:dbl)  [unwired: 1 in]
  n83 = property class="Bool (strict)"(reference=w182) -> (reference out=w184:refnum<vi>, error out=w183:errorcluster, "Value"=w174:bool)  [unwired: 1 in]
  n84 = property class="Bool (strict)"(reference=w198) -> (reference out=w200:refnum<vi>, error out=w199:errorcluster, "Value"=w152:bool)  [unwired: 1 in]
  n85 = property class="Bool (strict)"(reference=w206) -> (reference out=w204:refnum<vi>, error out=w205:errorcluster, "Value"=w153:bool)  [unwired: 1 in]
  n86 = property class="Bool (strict)"(reference=w201) -> (reference out=w203:refnum<vi>, error out=w202:errorcluster, "Value"=w154:bool)  [unwired: 1 in]
  n87 = property class="Bool (strict)"(reference=w171) -> (reference out=w169:refnum<vi>, error out=w170:errorcluster, "Value"=w155:bool)  [unwired: 1 in]
  n88 = property class="DigNum (strict)"(reference=w424) -> (reference out=w422:refnum<vi>, error out=w423:errorcluster, "Value"=w421:dbl)  [unwired: 1 in]
  n89 = property class="DigNum (strict)"(reference=w394) -> (reference out=w313:refnum<vi>, error out=w395:errorcluster, "Value"=w396:dbl)  [unwired: 1 in]
  n90 = property class="DigNum (strict)"(reference=w372) -> (reference out=w373:refnum<vi>, error out=w371:errorcluster, "Value"=w370:dbl)  [unwired: 1 in]
  n91 = property class="DigNum (strict)"(reference=w367) -> (reference out=w360:refnum<vi>, error out=w368:errorcluster, "Value"=w369:dbl)  [unwired: 1 in]
  n92 = property class="DigNum (strict)"(reference=w417) -> (reference out=w419:refnum<vi>, error out=w418:errorcluster, "Value"=w420:dbl)  [unwired: 1 in]
  n93 = property class="DigNum (strict)"(reference=w409) -> (reference out=w411:refnum<vi>, error out=w410:errorcluster, "Value"=w412:dbl)  [unwired: 1 in]
  n94 = property class="DigNum (strict)"(reference=w408) -> (reference out=w401:refnum<vi>, error out=w407:errorcluster, "Value"=w406:dbl)  [unwired: 1 in]
  n95 = property class="DigNum (strict)"(reference=w400) -> (reference out=w398:refnum<vi>, error out=w399:errorcluster, "Value"=w397:dbl)  [unwired: 1 in]
  n96 = property class="DigNum (strict)"(reference=w391) -> (reference out=w390:refnum<vi>, error out=w392:errorcluster, "Value"=w393:dbl)  [unwired: 1 in]
  n97 = property class="DigNum (strict)"(reference=w388) -> (reference out=w389:refnum<vi>, error out=w387:errorcluster, "Value"=w386:dbl)  [unwired: 1 in]
  n98 = property class="DigNum (strict)"(reference=w383) -> (reference out=w382:refnum<vi>, error out=w384:errorcluster, "Value"=w385:dbl)  [unwired: 1 in]
  n99 = property class="DigNum (strict)"(reference=w380) -> (reference out=w381:refnum<vi>, error out=w379:errorcluster, "Value"=w378:dbl)  [unwired: 1 in]
  n100 = property class="DigNum (strict)"(reference=w416) -> (reference out=w414:refnum<vi>, error out=w415:errorcluster, "Value"=w413:dbl)  [unwired: 1 in]
  n101 = property class="DigNum (strict)"(reference=w402) -> (reference out=w404:refnum<vi>, error out=w403:errorcluster, "Value"=w405:dbl)  [unwired: 1 in]
  n102 = property class="DigNum (strict)"(reference=w46) -> (reference out=w48:refnum<vi>, error out=w47:errorcluster, "Value"=w41:dbl)  [unwired: 1 in]
  n103 = property class="DigNum (strict)"(reference=w51) -> (reference out=w49:refnum<vi>, error out=w50:errorcluster, "Value"=w42:dbl)  [unwired: 1 in]
  n104 = property class="DigNum (strict)"(reference=w45) -> (reference out=w43:refnum<vi>, error out=w44:errorcluster, "Value"=w40:dbl)  [unwired: 1 in]
  n105 = Select(t=1, s=w174, f=0) -> (s? t:f=w129:i32)
  n106 = Select(t=1, s=w94, f=0) -> (s? t:f=w95:i32)
  n107 = Select(t=1, s=w152, f=0) -> (s? t:f=w151:i32)
  n108 = Select(t=1, s=w93, f=0) -> (s? t:f=w96:i32)
  n109 = Select(t=1, s=w92, f=0) -> (s? t:f=w97:i32)
  n110 = Select(t=1, s=w153, f=0) -> (s? t:f=w150:i32)
  n111 = Select(t=1, s=w154, f=0) -> (s? t:f=w149:i32)
  n112 = Select(t=1, s=w62, f=0) -> (s? t:f=w61:i32)
  n113 = Close Reference(reference=w65, error in (no error)=w64) -> ()  [unwired: 1 out]
  n114 = Select(t=1, s=w99, f=0) -> (s? t:f=w100:i32)
  n115 = Close Reference(reference=w88, error in (no error)=w89) -> ()  [unwired: 1 out]
  n116 = Select(t=1, s=w147, f=0) -> (s? t:f=w146:i32)
  n117 = Close Reference(reference=w356, error in (no error)=w354) -> ()  [unwired: 1 out]
  n118 = Close Reference(reference=w357, error in (no error)=w351) -> ()  [unwired: 1 out]
  n119 = Close Reference(reference=w158, error in (no error)=w157) -> ()  [unwired: 1 out]
  n120 = Select(t=1, s=w91, f=0) -> (s? t:f=w98:i32)
  n121 = Close Reference(reference=w73, error in (no error)=w74) -> ()  [unwired: 1 out]
  n122 = Close Reference(reference=w69, error in (no error)=w68) -> ()  [unwired: 1 out]
  n123 = Close Reference(reference=w70, error in (no error)=w71) -> ()  [unwired: 1 out]
  n124 = Close Reference(reference=w78, error in (no error)=w77) -> ()  [unwired: 1 out]
  n125 = Select(t=1, s=w155, f=0) -> (s? t:f=w148:i32)
  n126 = Close Reference(reference=w346, error in (no error)=w348) -> ()  [unwired: 1 out]
  n127 = Close Reference(reference=w339, error in (no error)=w341) -> ()  [unwired: 1 out]
  n128 = Close Reference(reference=w300, error in (no error)=w298) -> ()  [unwired: 1 out]
  n129 = Close Reference(reference=w293, error in (no error)=w295) -> ()  [unwired: 1 out]
  n130 = Close Reference(reference=w292, error in (no error)=w290) -> ()  [unwired: 1 out]
  n131 = Close Reference(reference=w285, error in (no error)=w287) -> ()  [unwired: 1 out]
  n132 = Close Reference(reference=w213, error in (no error)=w211) -> ()  [unwired: 1 out]
  n133 = Close Reference(reference=w214, error in (no error)=w216) -> ()  [unwired: 1 out]
  n134 = Close Reference(reference=w221, error in (no error)=w219) -> ()  [unwired: 1 out]
  n135 = Close Reference(reference=w178, error in (no error)=w176) -> ()  [unwired: 1 out]
  n136 = Close Reference(reference=w184, error in (no error)=w183) -> ()  [unwired: 1 out]
  n137 = Close Reference(reference=w186, error in (no error)=w188) -> ()  [unwired: 1 out]
  n138 = Close Reference(reference=w193, error in (no error)=w191) -> ()  [unwired: 1 out]
  n139 = Close Reference(reference=w194, error in (no error)=w196) -> ()  [unwired: 1 out]
  n140 = Close Reference(reference=w200, error in (no error)=w199) -> ()  [unwired: 1 out]
  n141 = Close Reference(reference=w204, error in (no error)=w205) -> ()  [unwired: 1 out]
  n142 = Close Reference(reference=w203, error in (no error)=w202) -> ()  [unwired: 1 out]
  n143 = Close Reference(reference=w169, error in (no error)=w170) -> ()  [unwired: 1 out]
  n144 = Close Reference(reference=w105, error in (no error)=w104) -> ()  [unwired: 1 out]
  n145 = Close Reference(reference=w338, error in (no error)=w344) -> ()  [unwired: 1 out]
  n146 = Close Reference(reference=w185, error in (no error)=w180) -> ()  [unwired: 1 out]
  n147 = Close Reference(reference=w132, error in (no error)=w133) -> ()  [unwired: 1 out]
  n148 = Close Reference(reference=w374, error in (no error)=w376) -> ()  [unwired: 1 out]
  n149 = Close Reference(reference=w359, error in (no error)=w362) -> ()  [unwired: 1 out]
  n150 = Close Reference(reference=w358, error in (no error)=w365) -> ()  [unwired: 1 out]
  n151 = Close Reference(reference=w422, error in (no error)=w423) -> ()  [unwired: 1 out]
  n152 = Close Reference(reference=w313, error in (no error)=w395) -> ()  [unwired: 1 out]
  n153 = Close Reference(reference=w373, error in (no error)=w371) -> ()  [unwired: 1 out]
  n154 = Close Reference(reference=w360, error in (no error)=w368) -> ()  [unwired: 1 out]
  n155 = Close Reference(reference=w419, error in (no error)=w418) -> ()  [unwired: 1 out]
  n156 = Close Reference(reference=w411, error in (no error)=w410) -> ()  [unwired: 1 out]
  n157 = Close Reference(reference=w401, error in (no error)=w407) -> ()  [unwired: 1 out]
  n158 = Close Reference(reference=w398, error in (no error)=w399) -> ()  [unwired: 1 out]
  n159 = Close Reference(reference=w390, error in (no error)=w392) -> ()  [unwired: 1 out]
  n160 = Close Reference(reference=w389, error in (no error)=w387) -> ()  [unwired: 1 out]
  n161 = Close Reference(reference=w382, error in (no error)=w384) -> ()  [unwired: 1 out]
  n162 = Close Reference(reference=w381, error in (no error)=w379) -> ()  [unwired: 1 out]
  n163 = Close Reference(reference=w414, error in (no error)=w415) -> ()  [unwired: 1 out]
  n164 = Close Reference(reference=w404, error in (no error)=w403) -> ()  [unwired: 1 out]
  n165 = Close Reference(reference=w48, error in (no error)=w47) -> ()  [unwired: 1 out]
  n166 = Close Reference(reference=w49, error in (no error)=w50) -> ()  [unwired: 1 out]
  n167 = Close Reference(reference=w43, error in (no error)=w44) -> ()  [unwired: 1 out]
  n168 = Number To Fractional String(number=w61, precision (6)=w60) -> (F-format string=w54:string)  [unwired: 2 in]
  n169 = Number To Fractional String(number=w95, precision (6)=w60) -> (F-format string=w59:string)  [unwired: 2 in]
  n170 = Number To Fractional String(number=w96, precision (6)=w60) -> (F-format string=w58:string)  [unwired: 2 in]
  n171 = Number To Fractional String(number=w97, precision (6)=w60) -> (F-format string=w57:string)  [unwired: 2 in]
  n172 = Number To Fractional String(number=w98, precision (6)=w60) -> (F-format string=w56:string)  [unwired: 2 in]
  n173 = Number To Fractional String(number=w100, precision (6)=w60) -> (F-format string=w55:string)  [unwired: 2 in]
  n174 = Number To Fractional String(number=w340, precision (6)=w60) -> (F-format string=w315:string)  [unwired: 2 in]
  n175 = Number To Fractional String(number=w299, precision (6)=w60) -> (F-format string=w284:string)  [unwired: 2 in]
  n176 = Number To Fractional String(number=w294, precision (6)=w60) -> (F-format string=w283:string)  [unwired: 2 in]
  n177 = Number To Fractional String(number=w291, precision (6)=w60) -> (F-format string=w282:string)  [unwired: 2 in]
  n178 = Number To Fractional String(number=w286, precision (6)=w60) -> (F-format string=w281:string)  [unwired: 2 in]
  n179 = Number To Fractional String(number=w212, precision (6)=w60) -> (F-format string=w209:string)  [unwired: 2 in]
  n180 = Number To Fractional String(number=w215, precision (6)=w60) -> (F-format string=w208:string)  [unwired: 2 in]
  n181 = Number To Fractional String(number=w220, precision (6)=w60) -> (F-format string=w207:string)  [unwired: 2 in]
  n182 = Number To Fractional String(number=w129, precision (6)=w60) -> (F-format string=w143:string)  [unwired: 2 in]
  n183 = Number To Fractional String(number=w187, precision (6)=w60) -> (F-format string=w142:string)  [unwired: 2 in]
  n184 = Number To Fractional String(number=w192, precision (6)=w60) -> (F-format string=w141:string)  [unwired: 2 in]
  n185 = Number To Fractional String(number=w195, precision (6)=w60) -> (F-format string=w140:string)  [unwired: 2 in]
  n186 = Number To Fractional String(number=w151, precision (6)=w60) -> (F-format string=w139:string)  [unwired: 2 in]
  n187 = Number To Fractional String(number=w150, precision (6)=w60) -> (F-format string=w138:string)  [unwired: 2 in]
  n188 = Number To Fractional String(number=w149, precision (6)=w60) -> (F-format string=w137:string)  [unwired: 2 in]
  n189 = Number To Fractional String(number=w148, precision (6)=w60) -> (F-format string=w136:string)  [unwired: 2 in]
  n190 = Number To Fractional String(number=w146, precision (6)=w60) -> (F-format string=w135:string)  [unwired: 2 in]
  n191 = Number To Fractional String(number=w421, precision (6)=w60) -> (F-format string=w336:string)  [unwired: 2 in]
  n192 = Number To Fractional String(number=w420, precision (6)=w60) -> (F-format string=w335:string)  [unwired: 2 in]
  n193 = Number To Fractional String(number=w412, precision (6)=w60) -> (F-format string=w334:string)  [unwired: 2 in]
  n194 = Number To Fractional String(number=w413, precision (6)=w60) -> (F-format string=w333:string)  [unwired: 2 in]
  n195 = Number To Fractional String(number=w406, precision (6)=w60) -> (F-format string=w332:string)  [unwired: 2 in]
  n196 = Number To Fractional String(number=w405, precision (6)=w60) -> (F-format string=w331:string)  [unwired: 2 in]
  n197 = Number To Fractional String(number=w396, precision (6)=w60) -> (F-format string=w330:string)  [unwired: 2 in]
  n198 = Number To Fractional String(number=w397, precision (6)=w60) -> (F-format string=w329:string)  [unwired: 2 in]
  n199 = Number To Fractional String(number=w393, precision (6)=w60) -> (F-format string=w328:string)  [unwired: 2 in]
  n200 = Number To Fractional String(number=w386, precision (6)=w60) -> (F-format string=w327:string)  [unwired: 2 in]
  n201 = Number To Fractional String(number=w385, precision (6)=w60) -> (F-format string=w326:string)  [unwired: 2 in]
  n202 = Number To Fractional String(number=w378, precision (6)=w60) -> (F-format string=w325:string)  [unwired: 2 in]
  n203 = Number To Fractional String(number=w377, precision (6)=w60) -> (F-format string=w324:string)  [unwired: 2 in]
  n204 = Number To Fractional String(number=w370, precision (6)=w60) -> (F-format string=w323:string)  [unwired: 2 in]
  n205 = Number To Fractional String(number=w369, precision (6)=w60) -> (F-format string=w322:string)  [unwired: 2 in]
  n206 = Number To Fractional String(number=w363, precision (6)=w60) -> (F-format string=w321:string)  [unwired: 2 in]
  n207 = Number To Fractional String(number=w364, precision (6)=w60) -> (F-format string=w320:string)  [unwired: 2 in]
  n208 = Number To Fractional String(number=w353, precision (6)=w60) -> (F-format string=w319:string)  [unwired: 2 in]
  n209 = Number To Fractional String(number=w352, precision (6)=w60) -> (F-format string=w318:string)  [unwired: 2 in]
  n210 = Number To Fractional String(number=w347, precision (6)=w60) -> (F-format string=w317:string)  [unwired: 2 in]
  n211 = Number To Fractional String(number=w345, precision (6)=w60) -> (F-format string=w316:string)  [unwired: 2 in]
  n212 = Number To Fractional String(number=w177, precision (6)=w60) -> (F-format string=w145:string)  [unwired: 2 in]
  n213 = Number To Fractional String(number=w179, precision (6)=w60) -> (F-format string=w144:string)  [unwired: 2 in]
  n214 = Number To Fractional String(number=w106, precision (6)=w60) -> (F-format string=w102:string)  [unwired: 2 in]
  n215 = Number To Fractional String(number=w131, precision (6)=w60) -> (F-format string=w130:string)  [unwired: 2 in]
  n216 = Number To Fractional String(number=w42) -> (F-format string=w39:string)  [unwired: 3 in]
  n217 = Number To Fractional String(number=w41) -> (F-format string=w38:string)  [unwired: 3 in]
  n218 = Number To Fractional String(number=w40) -> (F-format string=w37:string)  [unwired: 3 in]
  n219 = Insert Into Array(array=string[] [], new element #1=w336, new element #2=w335, new element #3=w334, new element #4=w333, new element #5=w332, new element #6=w331, new element #7=w330, new element #8=w329, new element #9=w328, new element #10=w327, new element #11=w326, new element #12=w325, new element #13=w324, new element #14=w323, new element #15=w322, new element #16=w321, new element #17=w320, new element #18=w319, new element #19=w318, new element #20=w317, new element #21=w316, new element #22=w315, new element #23=w284, new element #24=w283, new element #25=w282, new element #26=w281, new element #27=w209, new element #28=w208, new element #29=w207, new element #30=w145, new element #31=w144, new element #32=w143, new element #33=w142, new element #34=w141, new element #35=w140, new element #36=w139, new element #37=w138, new element #38=w137, new element #39=w136, new element #40=w135, new element #41=w130, new element #42=w102, new element #43=w59, new element #44=w58, new element #45=w57, new element #46=w56, new element #47=w55, new element #48=w54, new element #49=w39, new element #50=w38, new element #51=w37) -> (w314:string[])  [unwired: 1 in]
  n220 = for {
    tunnel: w432 -> [w444]
    tunnel: "CONFIG PARAMETER" ("WRITE /READ SECTION") -> [w443]
    tunnel: [w442] -> w430
    tunnel: string[] ["Sway PPR", "Sway Pitch", "Surge PPR", "Surge Pitch", "Heave PPR", "Heave Pitch", "Heave distance (mm)", "Surge distance (mm)", "Sway distance (mm)", "DataSavingLoopDelay(ms)", "Acoustic Emission:", "RotHomeSurgeOffsetCounts", "RotHomeSwayOffsetCounts", "TracHomeSurgeOffsetCounts 20MM", "TracHomeSwayOffsetCounts 20MM", "TracHomeSurgeOffsetCounts 10MM", "TracHomeSwayOffsetCounts 10MM", "LRMHomeSurgeOffsetCounts", "LRMHomeSwayOffsetCounts", "Filter% ", "Filter% 2", "SAMPLES", "Heave Loop Delay", "Heave PID Speed", "Surge Jog Speed", "Heave Jog Speed", "Sway Loop Delay", "Sway Pid Speed", "Sway Jog Speed", "Depth Trip Value", "Load Trip Value", "Depth Trip Enable", "Cyclic FF Trip Value", "FF Trip Value", "Cyclic Cof Trip Value", "Cyclic FF Trip Enable", "FF Trip Enable", "Cof Trip Enable", "Load Trip Enable", "Cyclic Cof Trip Enable", "COF TRIP VALUE", "JOG TRIP LOAD VALUE (N)", "ROTARY VERTICAL", "TRACTION", "SCRATCH", "LRM CAM", "SWAY LRM", "ROTARY HORIZONTAL", "SURGE SPEED", "SURGE BACKWARD COUNT", "SURGE FORWARD COUNT"] -> [w440] mode=indexing
    tunnel: w314 -> [w438] mode=indexing
    n221 = call "CONFIG FILE MAIN Unitest.vi"("WRITE /READ SECTION"=w443, "WRITE KEY"=w440, "WRITE VALUE"=w438, "error in"=w444, "PARAMETER/CONFIG"=TRUE, "Config Enum"=Config_file__FGV_Unitest_enum."WRITE") -> ("error out"=w442:errorcluster)  [unwired: 12 in, 1 out]
  }
  n222 = Unbundle By Name("main ref") -> ("About Screen.Humidity Port:"=w311:refnum<vi>)
  n223 = Unbundle By Name("main ref") -> ("About Screen.Temp Modbus:"=w306:refnum<vi>)
  n224 = Unbundle By Name("main ref") -> ("About Screen.ECR Port:"=w302:refnum<vi>)
  n225 = Unbundle By Name("main ref") -> ("New PID LOGIC.PID SDelay"=w276:refnum<vi>)
  n226 = Unbundle By Name("main ref") -> ("New PID LOGIC.Kp"=w275:refnum<vi>)
  n227 = Unbundle By Name("main ref") -> ("New PID LOGIC.Ki"=w270:refnum<vi>)
  n228 = Unbundle By Name("main ref") -> ("New PID LOGIC.Kd"=w269:refnum<vi>)
  n229 = Unbundle By Name("main ref") -> ("New PID LOGIC.Deadband"=w265:refnum<vi>)
  n230 = Unbundle By Name("main ref") -> ("New PID LOGIC.pct_scale"=w264:refnum<vi>)
  n231 = Unbundle By Name("main ref") -> ("New PID LOGIC.Init Step"=w261:refnum<vi>)
  n232 = Unbundle By Name("main ref") -> ("New PID LOGIC.i_limit"=w260:refnum<vi>)
  n233 = Unbundle By Name("main ref") -> ("New PID LOGIC.Max Step Linit"=w257:refnum<vi>)
  n234 = Unbundle By Name("main ref") -> ("New PID LOGIC.Max_pos_limit"=w255:refnum<vi>)
  n235 = Unbundle By Name("main ref") -> ("New PID LOGIC.Min_pos_limit"=w254:refnum<vi>)
  n236 = Unbundle By Name("main ref") -> ("New PID LOGIC.dynamic_spindle_noise_scalar"=w117:refnum<vi>)
  n237 = Unbundle By Name("main ref") -> ("New PID LOGIC.min_deadband_floor"=w112:refnum<vi>)
  n238 = property class="VISAName"(reference=w311) -> (reference out=w309:refnum<vi>, error out=w310:errorcluster, "Value"=w305:refnum<visa-resource-name>)  [unwired: 1 in]
  n239 = property class="VISAName"(reference=w306) -> (reference out=w308:refnum<vi>, error out=w307:errorcluster, "Value"=w304:refnum<visa-resource-name>)  [unwired: 1 in]
  n240 = Unbundle By Name("main ref") -> ("New PID LOGIC.min_finetune_floor"=w115:refnum<vi>)
  n241 = Unbundle By Name("main ref") -> ("New PID LOGIC.filter_alpha"=w118:refnum<vi>)
  n242 = property class="VISAName"(reference=w302) -> (reference out=w301:refnum<vi>, error out=w303:errorcluster, "Value"=w1:refnum<visa-resource-name>)  [unwired: 1 in]
  n243 = Close Reference(reference=w309, error in (no error)=w310) -> ()  [unwired: 1 out]
  n244 = Close Reference(reference=w308, error in (no error)=w307) -> ()  [unwired: 1 out]
  n245 = Close Reference(reference=w301, error in (no error)=w303) -> ()  [unwired: 1 out]
  n246 = property class="DigNum (strict)"(reference=w276) -> (reference out=w278:refnum<vi>, error out=w277:errorcluster, "Value"=w245:dbl)  [unwired: 1 in]
  n247 = property class="DigNum (strict)"(reference=w275) -> (reference out=w273:refnum<vi>, error out=w274:errorcluster, "Value"=w244:dbl)  [unwired: 1 in]
  n248 = property class="DigNum (strict)"(reference=w270) -> (reference out=w272:refnum<vi>, error out=w271:errorcluster, "Value"=w243:dbl)  [unwired: 1 in]
  n249 = property class="DigNum (strict)"(reference=w269) -> (reference out=w267:refnum<vi>, error out=w268:errorcluster, "Value"=w242:dbl)  [unwired: 1 in]
  n250 = property class="DigNum (strict)"(reference=w265) -> (reference out=w251:refnum<vi>, error out=w266:errorcluster, "Value"=w241:dbl)  [unwired: 1 in]
  n251 = property class="DigNum (strict)"(reference=w264) -> (reference out=w252:refnum<vi>, error out=w263:errorcluster, "Value"=w240:dbl)  [unwired: 1 in]
  n252 = property class="DigNum (strict)"(reference=w261) -> (reference out=w250:refnum<vi>, error out=w262:errorcluster, "Value"=w239:dbl)  [unwired: 1 in]
  n253 = property class="DigNum (strict)"(reference=w260) -> (reference out=w249:refnum<vi>, error out=w259:errorcluster, "Value"=w238:dbl)  [unwired: 1 in]
  n254 = property class="DigNum (strict)"(reference=w257) -> (reference out=w248:refnum<vi>, error out=w258:errorcluster, "Value"=w237:dbl)  [unwired: 1 in]
  n255 = property class="DigNum (strict)"(reference=w255) -> (reference out=w247:refnum<vi>, error out=w256:errorcluster, "Value"=w236:dbl)  [unwired: 1 in]
  n256 = property class="DigNum (strict)"(reference=w254) -> (reference out=w246:refnum<vi>, error out=w253:errorcluster, "Value"=w235:dbl)  [unwired: 1 in]
  n257 = property class="DigNum (strict)"(reference=w112) -> (reference out=w120:refnum<vi>, error out=w113:errorcluster, "Value"=w124:dbl)  [unwired: 1 in]
  n258 = property class="DigNum (strict)"(reference=w115) -> (reference out=w121:refnum<vi>, error out=w114:errorcluster, "Value"=w125:dbl)  [unwired: 1 in]
  n259 = property class="DigNum (strict)"(reference=w117) -> (reference out=w122:refnum<vi>, error out=w116:errorcluster, "Value"=w126:dbl)  [unwired: 1 in]
  n260 = property class="DigNum (strict)"(reference=w118) -> (reference out=w123:refnum<vi>, error out=w119:errorcluster, "Value"=w127:dbl)  [unwired: 1 in]
  n261 = Insert Into Array(array=string[] [], new element #1=w305, new element #2=w304, new element #3=w1) -> (w426:string[])  [unwired: 1 in]
  n262 = for {
    tunnel: w430 -> [w451]
    tunnel: "COM PORT" ("WRITE /READ SECTION") -> [w450]
    tunnel: [w449] -> w279
    tunnel: string[] ["HUMIDITY PORT", "TEMP MODBUS", "ECR PORT"] -> [w447] mode=indexing
    tunnel: w426 -> [w446] mode=indexing
    n263 = call "CONFIG FILE MAIN Unitest.vi"("WRITE /READ SECTION"=w450, "WRITE KEY"=w447, "WRITE VALUE"=w446, "error in"=w451, "PARAMETER/CONFIG"=TRUE, "Config Enum"=Config_file__FGV_Unitest_enum."WRITE") -> ("error out"=w449:errorcluster)  [unwired: 12 in, 1 out]
  }
  n264 = Close Reference(reference=w278, error in (no error)=w277) -> ()  [unwired: 1 out]
  n265 = Close Reference(reference=w273, error in (no error)=w274) -> ()  [unwired: 1 out]
  n266 = Close Reference(reference=w272, error in (no error)=w271) -> ()  [unwired: 1 out]
  n267 = Close Reference(reference=w267, error in (no error)=w268) -> ()  [unwired: 1 out]
  n268 = Close Reference(reference=w251, error in (no error)=w266) -> ()  [unwired: 1 out]
  n269 = Close Reference(reference=w252, error in (no error)=w263) -> ()  [unwired: 1 out]
  n270 = Close Reference(reference=w250, error in (no error)=w262) -> ()  [unwired: 1 out]
  n271 = Close Reference(reference=w249, error in (no error)=w259) -> ()  [unwired: 1 out]
  n272 = Close Reference(reference=w248, error in (no error)=w258) -> ()  [unwired: 1 out]
  n273 = Close Reference(reference=w247, error in (no error)=w256) -> ()  [unwired: 1 out]
  n274 = Close Reference(reference=w246, error in (no error)=w253) -> ()  [unwired: 1 out]
  n275 = Close Reference(reference=w120, error in (no error)=w113) -> ()  [unwired: 1 out]
  n276 = Close Reference(reference=w121, error in (no error)=w114) -> ()  [unwired: 1 out]
  n277 = Close Reference(reference=w122, error in (no error)=w116) -> ()  [unwired: 1 out]
  n278 = Close Reference(reference=w123, error in (no error)=w119) -> ()  [unwired: 1 out]
  n279 = Number To Fractional String(number=w245, precision (6)=w111) -> (F-format string=w233:string)  [unwired: 2 in]
  n280 = Number To Fractional String(number=w244, precision (6)=w111) -> (F-format string=w232:string)  [unwired: 2 in]
  n281 = Number To Fractional String(number=w243, precision (6)=w111) -> (F-format string=w231:string)  [unwired: 2 in]
  n282 = Number To Fractional String(number=w242, precision (6)=w111) -> (F-format string=w230:string)  [unwired: 2 in]
  n283 = Number To Fractional String(number=w241, precision (6)=w111) -> (F-format string=w229:string)  [unwired: 2 in]
  n284 = Number To Fractional String(number=w240, precision (6)=w111) -> (F-format string=w228:string)  [unwired: 2 in]
  n285 = Number To Fractional String(number=w239, precision (6)=w111) -> (F-format string=w227:string)  [unwired: 2 in]
  n286 = Number To Fractional String(number=w238, precision (6)=w111) -> (F-format string=w226:string)  [unwired: 2 in]
  n287 = Number To Fractional String(number=w237, precision (6)=w111) -> (F-format string=w225:string)  [unwired: 2 in]
  n288 = Number To Fractional String(number=w236, precision (6)=w111) -> (F-format string=w224:string)  [unwired: 2 in]
  n289 = Number To Fractional String(number=w235, precision (6)=w111) -> (F-format string=w223:string)  [unwired: 2 in]
  n290 = Number To Fractional String(number=w124, precision (6)=w111) -> (F-format string=w110:string)  [unwired: 2 in]
  n291 = Number To Fractional String(number=w125, precision (6)=w111) -> (F-format string=w109:string)  [unwired: 2 in]
  n292 = Number To Fractional String(number=w126, precision (6)=w111) -> (F-format string=w108:string)  [unwired: 2 in]
  n293 = Number To Fractional String(number=w127, precision (6)=w111) -> (F-format string=w107:string)  [unwired: 2 in]
  n294 = Insert Into Array(array=string[] [], new element #1=w233, new element #2=w232, new element #3=w231, new element #4=w230, new element #5=w229, new element #6=w228, new element #7=w227, new element #8=w226, new element #9=w225, new element #10=w224, new element #11=w223, new element #12=w110, new element #13=w109, new element #14=w108, new element #15=w107) -> (w222:string[])  [unwired: 1 in]
  n295 = for {
    tunnel: w279 -> [w458]
    tunnel: "NEW PID PARAMETERS" ("WRITE /READ SECTION") -> [w457]
    tunnel: [w456] -> w34
    tunnel: string[] ["PID DELAY (sec)", "Kp", "Ki", "Kd", "Deaadband", "pct_scale", "Init_step", "i_limit", "Max Step Limit", "Min_pos_limit", "Max_pos_limit", "Fine_tune_zone", "min_deadband_floor", "min_finetune_floor", "dynamic_spindle_noise_scalar", "filter_alpha"] -> [w454] mode=indexing
    tunnel: w222 -> [w452] mode=indexing
    n296 = call "CONFIG FILE MAIN Unitest.vi"("WRITE /READ SECTION"=w457, "WRITE KEY"=w454, "WRITE VALUE"=w452, "error in"=w458, "PARAMETER/CONFIG"=TRUE, "Config Enum"=Config_file__FGV_Unitest_enum."WRITE") -> ("error out"=w456:errorcluster)  [unwired: 12 in, 1 out]
  }
  n297 = Unbundle By Name("main ref") -> ("ABOUT.version"=w28:refnum<vi>)
  n298 = Unbundle By Name("main ref") -> ("ABOUT.Operating System"=w27:refnum<vi>)
  n299 = Unbundle By Name("main ref") -> ("ABOUT.Version"=w21:refnum<vi>)
  n300 = Unbundle By Name("main ref") -> ("ABOUT.Workorder"=w22:refnum<vi>)
  n301 = Unbundle By Name("main ref") -> ("ABOUT.Runtime"=w12:refnum<vi>)
  n302 = Unbundle By Name("main ref") -> ("ABOUT.Instrument Serial"=w13:refnum<vi>)
  n303 = Unbundle By Name("main ref") -> ("ABOUT.Firmware Version"=w16:refnum<vi>)
  n304 = property class="Str"(reference=w28) -> (reference out=w30:refnum<vi>, error out=w29:errorcluster, "Value"=w8:string)  [unwired: 1 in]
  n305 = property class="Str"(reference=w27) -> (reference out=w25:refnum<vi>, error out=w26:errorcluster, "Value"=w7:string)  [unwired: 1 in]
  n306 = property class="Str"(reference=w21) -> (reference out=w19:refnum<vi>, error out=w20:errorcluster, "Value"=w6:string)  [unwired: 1 in]
  n307 = property class="Str"(reference=w22) -> (reference out=w24:refnum<vi>, error out=w23:errorcluster, "Value"=w5:string)  [unwired: 1 in]
  n308 = property class="Str"(reference=w12) -> (reference out=w10:refnum<vi>, error out=w11:errorcluster, "Value"=w4:string)  [unwired: 1 in]
  n309 = property class="Str"(reference=w16) -> (reference out=w18:refnum<vi>, error out=w17:errorcluster, "Value"=w2:string)  [unwired: 1 in]
  n310 = property class="Str"(reference=w13) -> (reference out=w15:refnum<vi>, error out=w14:errorcluster, "Value"=w3:string)  [unwired: 1 in]
  n311 = Close Reference(reference=w30, error in (no error)=w29) -> ()  [unwired: 1 out]
  n312 = Close Reference(reference=w25, error in (no error)=w26) -> ()  [unwired: 1 out]
  n313 = Close Reference(reference=w19, error in (no error)=w20) -> ()  [unwired: 1 out]
  n314 = Close Reference(reference=w24, error in (no error)=w23) -> ()  [unwired: 1 out]
  n315 = Close Reference(reference=w10, error in (no error)=w11) -> ()  [unwired: 1 out]
  n316 = Close Reference(reference=w15, error in (no error)=w14) -> ()  [unwired: 1 out]
  n317 = Close Reference(reference=w18, error in (no error)=w17) -> ()  [unwired: 1 out]
  n318 = Insert Into Array(array=string[] [], new element #1=w8, new element #2=w7, new element #3=w6, new element #4=w5, new element #5=w4, new element #6=w3, new element #7=w2) -> (w31:string[])  [unwired: 1 in]
  n319 = for {
    tunnel: "ABOUT SCREEN" ("WRITE /READ SECTION") -> [w465]
    tunnel: [w464] -> w33
    tunnel: string[] ["version", "Operating System", "Version", "Workorder", "runtime", "Instrument Serial Number", "Firmware version"] -> [w462] mode=indexing
    tunnel: w34 -> [w460]
    tunnel: w31 -> [w459] mode=indexing
    n320 = call "CONFIG FILE MAIN Unitest.vi"("WRITE /READ SECTION"=w465, "WRITE KEY"=w462, "WRITE VALUE"=w459, "error in"=w460, "PARAMETER/CONFIG"=TRUE, "Config Enum"=Config_file__FGV_Unitest_enum."WRITE") -> ("error out"=w464:errorcluster)  [unwired: 12 in, 1 out]
  }
  n321 = call "CONFIG FILE MAIN Unitest.vi"("error in"=w33, "Config Enum"=Config_file__FGV_Unitest_enum."CLOSE") -> ("error out"=→"error out":errorcluster)  [unwired: 16 in, 1 out]
